vi "Create CSI-2 Packet TDMS Files powered by aTTIS.vi"() -> ()   [LabVIEW 2025, in "GettingStarted_Gen_148X_Host.lvlib"]
uses:
  GettingStarted_Gen_148X_Host.lvlib
  Types/Frame Data Configuration.ctl
  <instrlib>/FlexRIO/CSI-2/v2/Common/Types/LLP Data Type.ctl
  Types/Frame Timing Configuration.ctl
  Common/GettingStarted_Common_148X_Host.lvlib
  <instrlib>/FlexRIO/CSI-2/v2/Common/NI CSI-2 API Common v2.lvlib
panel:
  out "subarray":u8[][](array[numeric])
  out "floor(x/y)":u32
  out "Actrual Frame":i32
  in  "Generate LLP Packet Offsets":bool=TRUE
  in  "Serial Input Channels":string[](array[string])=["SI0"]
  out "Actual Frame Rate (fps)":dbl
  in  "Frame Timing Configuration":T1={"desired frame rate (fps)"=30.0, "actual link data rate (B/s)"=385000000.0, "minimum delay between packets (cycles)"=500, "line blanking (cycles)"=1000} {"actual link data rate (B/s)" format="%_6p"; "line blanking (cycles)" format="%#.0f"}
  in  "Number of Frames":i32=10
  in  "Frame Data Configuration":T2={"pixel data type"=enum."RAW 12", "horizontal resolution"=1920, "vertical resolution"=1080, "virtual channel"=0.0, "include line sync packets"=FALSE}
  out "Error Out":errorcluster
  in  "TDMS File Directory":path
  # "Overview: Create sample TDMS files for use with the Generation Getting Started example.  \nInstructions: Visit https://ni.com/r/automotive-camera-module-ref for a detailed tutorial or use the basic instructions below.\n\n 1. Select the serial input channel names to use when creating the files.  The Generation Getting Started example expects the serial input channel number of the file to match the serial output channel number used to generate the data.\n 2. Select the destination directory for the created TDMS files.  Leave blank to use the \"TDMS Files\" directory in the same directory as this VI.\n 3. Select the number of frames to create. \n 4. Select the frame data configuration.  This determines what the frames will look like.  Each frame will be identical with the exception of the frame number.  Each line within a frame will be identical with the exception of the line number (if configured to send line sync packets).  The packet payload is a byte ramp; this is independent of the pixel data type.\n 5. Select the frame timing configuration.  This determines the timing of the individual packets.  The Actual Frame Rate (fps) indicator shows the frame rate of the generated data.  It is possible that this will be lower than the desired frame rate because the interpacket delay cycles and line blanking cycles  are priortized over the frame rate."
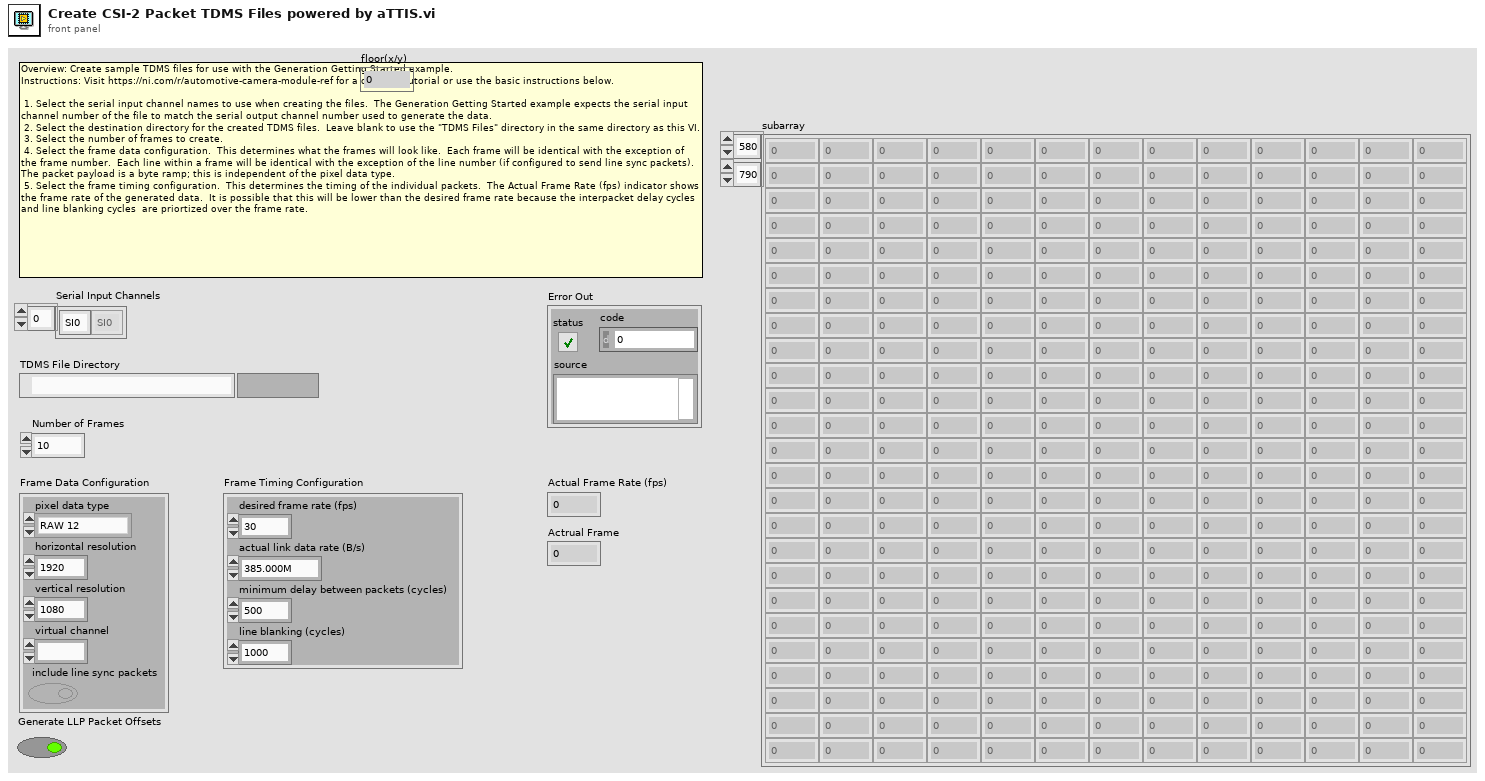
[diagram p1: front panel]
types:
  T1 = typedef "GettingStarted_Gen_148X_Host.lvlib/Frame Timing Configuration.ctl" = cluster{"desired frame rate (fps)":dbl, "actual link data rate (B/s)":dbl, "minimum delay between packets (cycles)":u64, "line blanking (cycles)":u64}
  T2 = typedef "GettingStarted_Gen_148X_Host.lvlib/Frame Data Configuration.ctl" = cluster{"pixel data type":T3, "horizontal resolution":u16, "vertical resolution":u16, "virtual channel":fxp<+,4,4>, "include line sync packets":bool}
  T3 = typedef "NI CSI-2 API Common v2.lvlib/LLP Data Type.ctl" = enum8{"Frame Start", "Frame End", "Line Start", "Line End", "End of Transmission", "Reserved 0", "Reserved 1", "Reserved 2", "Generic Short Packet 1", "Generic Short Packet 2", "Generic Short Packet 3", "Generic Short Packet 4", "Generic Short Packet 5", "Generic Short Packet 6", "Generic Short Packet 7", "Generic Short Packet 8", "Null", "Blanking Data", "Embedded 8-bit non Image Data", "Generic Long Packet 1", "Generic Long Packet 2", "Generic Long Packet 3", "Generic Long Packet 4", "Reserved 3", "YUV420 8-bit", "YUV420 10-bit", "Legacy YUV420 8-bit", "Reserved 4", "YUV420 8-bit Chroma Shifted", "YUV420 10-bit Chroma Shifted", "YUV422 8-bit", "YUV422 10-bit", "RGB444", "RGB555", "RGB565", "RGB666", "RGB888", "Reserved 5", "Reserved 6", "RAW 24", "RAW 6", "RAW 7", "RAW 8", "RAW 10", "RAW 12", "RAW 14", "RAW 16", "RAW 20", "User Defined 8-bit Data 1", "User Defined 8-bit Data 2", "User Defined 8-bit Data 3", "User Defined 8-bit Data 4", "User Defined 8-bit Data 5", "User Defined 8-bit Data 6", "User Defined 8-bit Data 7", "User Defined 8-bit Data 8", "USL Command", "Reserved 7", "Reserved 8", "Reserved 9", "Reserved 10", "Reserved 11", "Reserved 12", "LRTE EPD Spacer"}
  T4 = enum16{"open", "open or create", "create or replace", "create", "open (read-only)"}
  T5 = enum16{"big-endian, network order", "native, host order", "little-endian"}
  T6 = typedef "NI CSI-2 API Host v2.lvlib/Host LLP Packet.ctl" = cluster{"header":T7, "payload":u8[], "footer":T8}
  T7 = typedef "NI CSI-2 API FPGA v2.lvlib/LLP Packet Header.ctl" = cluster{"word count":u16, "ecc":fxp<+,6,6>, "vcx":fxp<+,2,2>, "data type":fxp<+,6,6>, "vc":fxp<+,2,2>}
  T8 = typedef "NI CSI-2 API FPGA v2.lvlib/LLP Packet Footer.ctl" = cluster{"crc":u16}
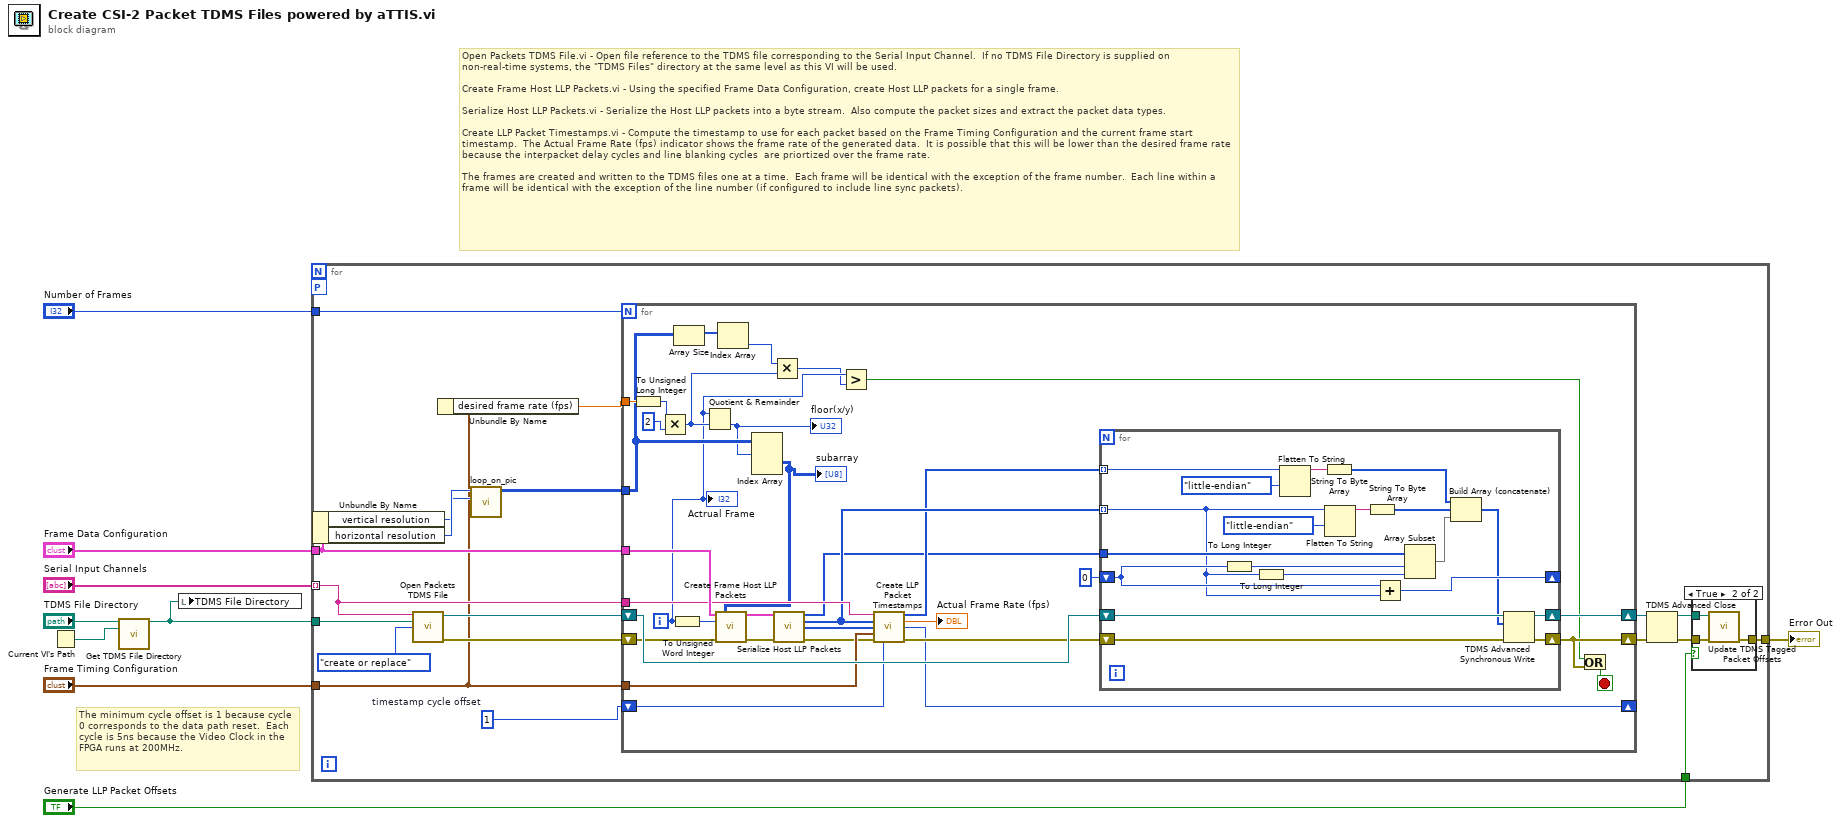
[diagram p0: block diagram]
diagram:
  # "The minimum cycle offset is 1 because cycle 0 corresponds to the data path reset.  Each cycle is 5ns because the Video Clock in the FPGA runs at 200MHz."
  # "Open Packets TDMS File.vi - Open file reference to the TDMS file corresponding to the Serial Input Channel.  If no TDMS File Directory is supplied on non-real-time systems, the \"TDMS Files\" directory at the same level as this VI will be used.\n\nCreate Frame Host LLP Packets.vi - Using the specified Frame Data Configuration, create Host LLP packets for a single frame.\n\nSerialize Host LLP Packets.vi - Serialize the Host LLP packets into a byte stream.  Also compute the packet sizes and extract the packet data types. \n\nCreate LLP Packet Timestamps.vi - Compute the timestamp to use for each packet based on the Frame Timing Configuration and the current frame start timestamp.  The Actual Frame Rate (fps) indicator shows the frame rate of the generated data.  It is possible that this will be lower than the desired frame rate because the interpacket delay cycles and line blanking cycles  are priortized over the frame rate.\n\nThe frames are created and written to the TDMS files one at a time.  Each frame will be identical with the exception of the frame number.  Each line within a frame will be identical with the exception of the line number (if configured to include line sync packets)."
  n1 = Current VI's Path() -> (path=w3:path)
  n2 = call "Get TDMS File Directory.vi"("tdms file directory in"="TDMS File Directory", "calling vi path"=w3) -> ("tdms file directory out"=w5:path)  [unwired: 13 in]
  n3 = local write "TDMS File Directory"(w5) -> ()
  n4 = for {
    tunnel: [w17] -> w2
    tunnel: "Frame Data Configuration" -> [w15]
    tunnel: "Number of Frames" -> [w28]
    tunnel: "Frame Timing Configuration" -> [w12]
    tunnel: w5 -> [w23]
    tunnel: "Serial Input Channels" -> [w24] mode=indexing
    workers-P: _ -> [_]
    tunnel: "Generate LLP Packet Offsets" -> [w16]
    w25 = u64 1  # timestamp cycle offset
    n5 = Unbundle By Name(w15) -> ("vertical resolution"=w13:u16, "horizontal resolution"=w14:u16)
    n6 = call "Open Packets TDMS File.vi"("serial input channel"=w24, "base tdms file path"=w23, "file operation type"=T4."create or replace") -> ("packets file ref"=w26:refnum<k34>, "error out"=w22:errorcluster)  [unwired: 11 in]
    n7 = Unbundle By Name(w12) -> ("desired frame rate (fps)"=w10:dbl)
    n8 = call "loop_on_pic.vi"("Y Resolution"=w13, "X Resolution"=w14) -> ("Image Pixels (U8)"=w11:u8[][][])  [unwired: 8 in, 1 out]
    n9 = for {
      N: w28 -> [_]
      tunnel: w15 -> [w64]
      tunnel: w24 -> [w62]
      shift-right: [w50] -> w27
      shift-left: w26 -> [w65]
      shift-right: [w59] -> _
      shift-left: w25 -> [w57]
      tunnel: w12 -> [w56]
      shift-right: [w39] -> w20
      shift-left: w22 -> [w63]
      tunnel: w11 -> [w43]
      tunnel: w10 -> [w46]
      i -> [w38]
      stop <- w35 stop-if-true
      n10 = To Unsigned Long Integer(number=w46) -> (unsigned 32bit integer=w45:u32)
      n11 = Multiply(x=w45, y=u32 2) -> (x*y=w41:u32)
      n12 = To Unsigned Word Integer(number=w38) -> (unsigned 16bit integer=w60:u16)
      n13 = Array Size(array=w43) -> (size(s)=w42:i32[])
      n14 = Quotient & Remainder(x=w38, y=w41) -> (floor(x/y)=w34:u32)  [unwired: 1 out]
      "floor(x/y)" <- w34
      n15 = Index Array(array=w42) -> (element=w40:i32)  [unwired: 1 in]
      n16 = Index Array(array=w43, index (dim 0)=w34) -> (element=w33:u8[][])  [unwired: 2 in]
      "subarray" <- w33
      n17 = call "Create Frame Host LLP Packets.vi"("frame configuration"=w64, "Array"=w33, "frame number"=w60, "error in (no error)"=w63) -> ("frame packets"=w55:T6[], "error out"=w54:errorcluster)  [unwired: 10 in]
      n18 = Multiply(x=w40, y=w41) -> (x*y=w37:u32)
      n19 = call "Serialize Host LLP Packets.vi"("host llp packets"=w55, "error in (no error)"=w54) -> ("packet bytes"=w48:u8[], "packet sizes"=w53:u32[], "packet data types"=w52:T3[], "error out"=w51:errorcluster)  [unwired: 10 in]
      n20 = Greater?(x=w38, y=w37) -> (0:w36:bool)
      n21 = call "Create LLP Packet Timestamps.vi"("serial input channel"=w62, "llp packet sizes"=w53, "packet data types"=w52, "frame timing configuration"=w56, "error in (no error)"=w51, "frame start timestamp"=w57) -> ("timestamps"=w49:u64[], "actual frame rate (fps)"=→"Actual Frame Rate (fps)":dbl, "next frame start timestamp"=w59:u64, "error out"=w61:errorcluster)  [unwired: 6 in]
      n22 = for {
        tunnel: w53 -> [w74] mode=indexing
        tunnel: w49 -> [w84] mode=indexing
        shift-right: [w68] -> w50
        shift-left: w65 -> [w69]
        shift-right: [w70] -> w39
        shift-left: w61 -> [w67]
        shift-right: [w81] -> _
        shift-left: u32 0 -> [w79]
        tunnel: w48 -> [w80]
        n23 = To Long Integer(number=w79) -> (32bit integer=w76:i32)
        n24 = To Long Integer(number=w74) -> (32bit integer=w75:i32)
        n25 = Flatten To String(anything=w84, byte order (0:big-endian, network order)=T5."little-endian") -> (data string=w83:string)  [unwired: 2 in, 2 out]
        n26 = String To Byte Array(string=w83) -> (unsigned byte array=w71:u8[])
        n27 = Flatten To String(anything=w74, byte order (0:big-endian, network order)=T5."little-endian") -> (data string=w82:string)  [unwired: 2 in, 2 out]
        n28 = String To Byte Array(string=w82) -> (unsigned byte array=w72:u8[])
        n29 = Add(x=w79, y=w74) -> (x+y=w81:u32)
        n30 = Array Subset(array=w80, index=w76, length=w75) -> (w73:u8[])
        n31 = Build Array (concatenate)(w71, w72, w73) -> (w66:u8[])
        n32 = TDMS Advanced Synchronous Write(8:w67, 10:w66, 11:w69) -> (0:w70:errorcluster, 3:w68:refnum<k34>)
      }
      n33 = Or(x=w36, y=w39) -> (x .or. y?=w35:bool)
      "Actrual Frame" <- w38
    }
    n34 = TDMS Advanced Close(8:w20, 11:w27) -> (0:w18:errorcluster, 3:w19:path)  [unwired: 2 in]
    n35 = case shown="True" w16 {
      tunnel: w19 -> [_ w32]
      tunnel: w18 -> [w29 w31]
      tunnel: [w29 w30] -> w17
      frame False {
      }
      frame True {
        n36 = call "Update TDMS Tagged Packet Offsets.vi"("llp tagged packet file path"=w32, "error in"=w31) -> ("error out"=w30:errorcluster)  [unwired: 12 in, 1 out]
      }
    }
  }
  "Error Out" <- w2
